vi "read_txt.vi"(8 "error in":errorcluster, 11 "file (use dialog)":path) -> (0 "error out":errorcluster, 3 "Array(lon, lat)":dbl[][](array[numeric]) format="%#.9g")   [LabVIEW 2020]
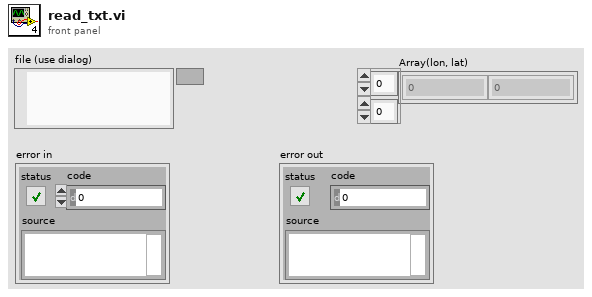
[diagram p1: front panel]
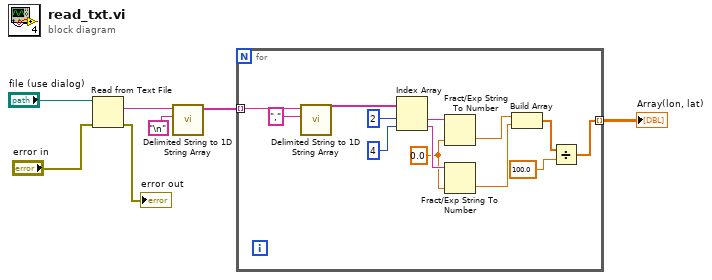
[diagram p0: block diagram]
diagram:
  n1 = Read from Text File(file (use dialog)="file (use dialog)", error in="error in") -> (text=w5:string, error out=→"error out":errorcluster)  [unwired: 2 in, 2 out]
  n2 = call <vilib>:"Delimited String to 1D String Array.vi"("delimiter"="\n", "delimited string"=w5) -> ("string array"=w3:string[])  [unwired: 9 in]
  n3 = for {
    tunnel: w3 -> [w20] mode=indexing
    tunnel: [w8] -> w2 mode=indexing
    w12 = 0.0 ("default (0 DBL)")
    n4 = call <vilib>:"Delimited String to 1D String Array.vi"("delimiter"=",", "delimited string"=w20) -> ("string array"=w18:string[])  [unwired: 9 in]
    n5 = Index Array(array=w18, index #1=2 ("index"), index #2=4 ("index")) -> (element #1=w15:string, element #2=w13:string)
    n6 = Fract/Exp String To Number(string=w15, default (0 dbl)=w12) -> (number=w14:dbl)  [unwired: 2 in, 1 out]
    n7 = Fract/Exp String To Number(string=w13, default (0 dbl)=w12) -> (number=w11:dbl)  [unwired: 2 in, 1 out]
    n8 = Build Array(w14, w11) -> (w10:dbl[])
    n9 = Divide(x=w10, y=100.0 ("default (0 DBL)")) -> (x/y=w8:dbl[])
  }
  "Array(lon, lat)" <- w2
